vi "mro_read_flat.vi"(7 "FilePath":string="FLAT_MIRAO_0229_01.mro", 8 "error in (no error)":errorcluster, 11 "status in":i32) -> (0 "error out":errorcluster, 1 "flat":dbl[](array[numeric]), 2 "return type":i8, 3 "status out":i32)   [LabVIEW 2011]
uses:
  mirao52e.dll
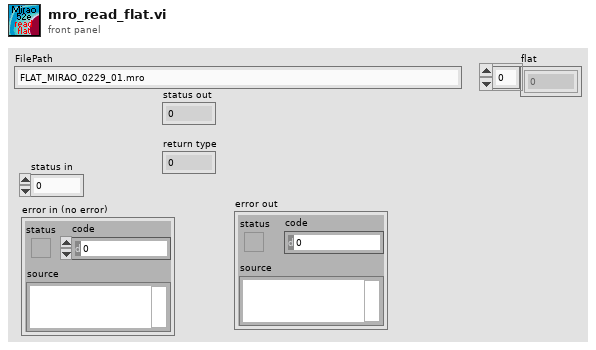
[diagram p1: front panel]
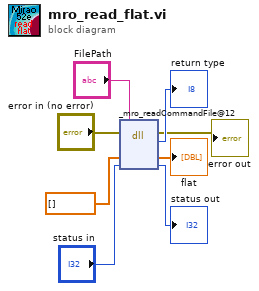
[diagram p0: block diagram]
diagram:
  n1 = dll-call lib="C:/Users/myerslab/workspace2/Mirao52J/labview/mirao52e.dll" fn="_mro_readCommandFile@12"(error in="error in (no error)", "FilePath"="FilePath", "command"=dbl[] [], "status"="status in") -> (error out=→"error out":errorcluster, "return type"=→"return type":i8, "command"=→"flat":dbl[], "status"=→"status out":i32)  [unwired: 3 in, 1 out]
